vi "PC_Consumer_DMA.vi"() -> ()   [LabVIEW 2019]
uses:
  <vilib>/FPGAPlugInAG/cRIO-9074/niLvFpga_Open_cRIO-9074.vi
  <vilib>/FPGAPlugInAG/cRIO-9074/niLvFpga_Reset_cRIO-9074.vi
  <vilib>/rvi/interface/common/niFpgaWaitOnOcc.vi
  <vilib>/Utility/error.llb/Error Cluster From Error Code.vi
  <vilib>/rvi/errors/niLvFpgaAdjustHostInterfaceError.vi
  <vilib>/FPGAPlugInAG/cRIO-9074/niLvFpga_Run_cRIO-9074.vi
  <vilib>/RVI Host/nirviSupport.llb/nirviErrorClusterFromErrorCode.vi
  FPGA_RW_Vars.vi
  <vilib>/FPGAPlugInAG/cRIO-9074/niLvFpga_Close_cRIO-9074.vi
  <vilib>/rvi/interface/nirviOpenFPGA/nirviOpenFPGA.xnode
  FPGA Bitfiles/bancadaamaciamen_FPGATarget_[FPGA]DeltaSigMa_JyyHRzhCmwA.lvbitx
  FPGA_DAQ_Int.vi
  <vilib>/rvi/interface/nirviMethod/nirviMethod.xnode
  <vilib>/rvi/interface/nirviReadWriteControl/nirviReadWriteControl.xnode
  <vilib>/rvi/interface/nirviCloseFPGA/nirviCloseFPGA.xnode
  <vilib>/rvi/errors/niLvFpgaMergeErrorWithErrorCode.vi
  <vilib>/rvi/interface/nirviMethod/StockFPGA_InlinedMethodWaitForSingleIRQ.vi
  <vilib>/FPGAPlugInAG/cRIO-9074/niLvFpga_WaitOnIrq_cRIO-9074.vi
  <vilib>/FPGAPlugInAG/cRIO-9074/niLvFpga_AcknowledgeIrq_cRIO-9074.vi
  <vilib>/FPGAPlugInAG/cRIO-9074/niLvFpga_ConfigureFifo_cRIO-9074.vi
  <vilib>/FPGAPlugInAG/cRIO-9074/niLvFpga_StartFifo_cRIO-9074.vi
  NiFpgaLv.dll
  <vilib>/FPGAPlugInAG/cRIO-9074/niLvFpga_ReadFifo_cRIO-9074.vi
  <vilib>/FPGAPlugInAG/cRIO-9074/niLvFpga_StopFifo_cRIO-9074.vi
panel:
  out "Vibração + Tensão":waveform(dbl)[](graph)
  in  "Reset Vibracão":bool caption="Reset"
  in  "Reset Tensão":bool caption="Reset"
  out "Gráfico Tensão":waveform(dbl)(graph)
  out "Gráfico Vibração":waveform(dbl)(graph)
  out "Reading?":bool
  out "Calibration Voltage (NI 9225)":cluster{"LSB Weight":dbl, "Offset":dbl}[](array[cluster])
  out "Calibration Vibration (NI 9234)":cluster{"LSB Weight":dbl, "Offset":dbl}[](array[cluster])
  out "Calibration Current (NI 9215)":cluster{"LSB Weight":dbl, "Offset":dbl}[](array[cluster])
  out "Temperature 2 (NI-9219)":T1
  out "Vibration (NI-9234)":cluster{"Vibration (CH1)":waveform(dbl)}
  out "Voltage (NI-9225)":cluster{"Voltage (CH0)":waveform(dbl)}
  out "Voltage (NI-9215)":cluster{"Voltage LEM (CH3)":waveform(dbl)}
  out "Temperature (NI-9219)":T1
  out "Waveform Volt":waveform(dbl)[](graph)
  out "Waveform Cur":waveform(dbl)[](graph)
  in  "ElementsPerCycle":u32=25600
  out "Waveform Vib":waveform(dbl)[](graph)
  out "Configuração realizada":bool
  out "Actual Depth":i32
  out "Requested Depth":i32
  out "Measurements per Cycle":i32
  in  "Stop":bool
  out "Error Out":errorcluster
  # "Configuração"
  # "Leitura"
  # "Sensores de Vibração"
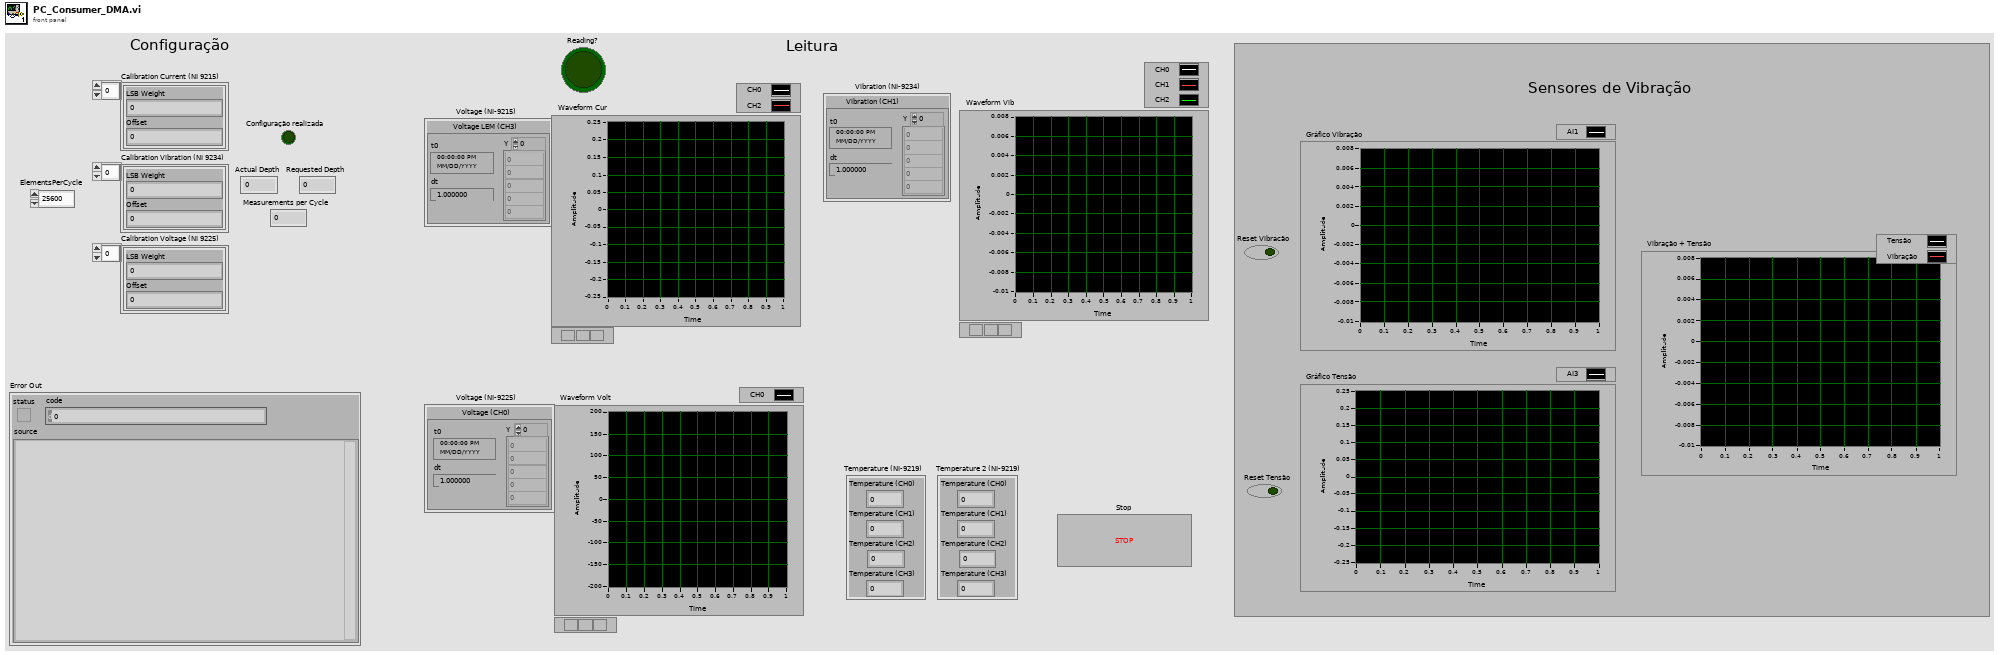
[diagram p1: front panel]
types:
  T1 = cluster{"Temperature (CH0)":dbl, "Temperature (CH1)":dbl, "Temperature (CH2)":dbl, "Temperature (CH3)":dbl}
  T2 = cluster{"Temperature (ºC)":dbl, "Temperature (ºC)":dbl, "Temperature (ºC)":dbl, "Temperature (ºC)":dbl}
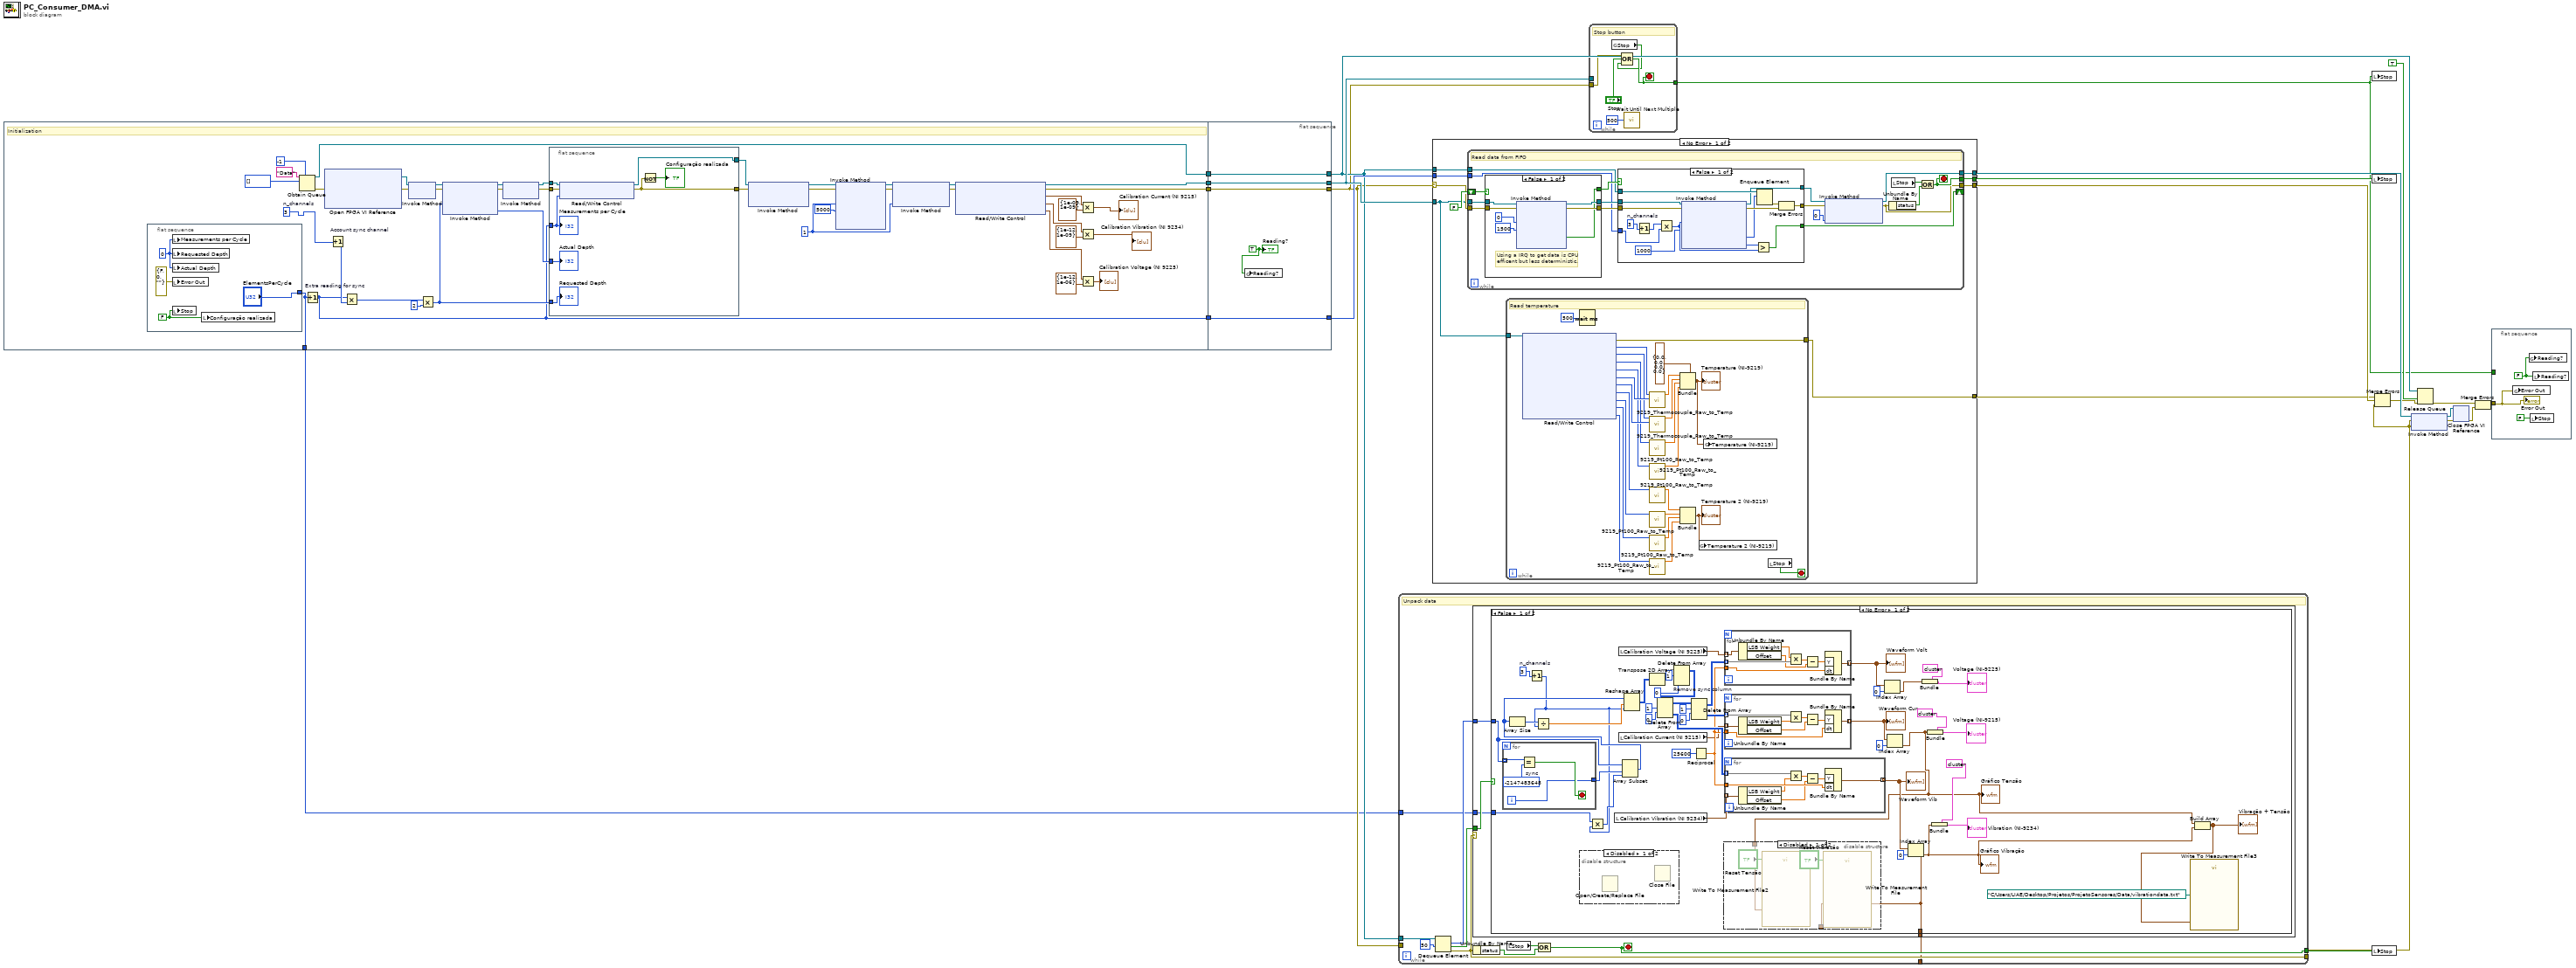
[diagram p0: block diagram]
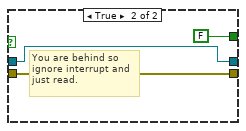
[diagram p6: hidden frame]
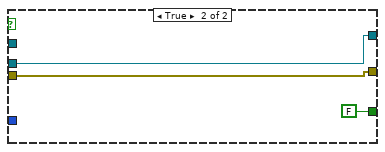
[diagram p7: hidden frame]
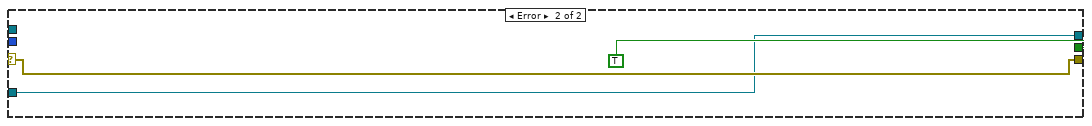
[diagram p8: hidden frame]
diagram:
  n1 = flat-sequence {
    tunnel: [w25] -> w5
    tunnel: [w39] -> w4
    tunnel: [w51] -> w3
    tunnel: [w38] -> w2
    tunnel: [w24] -> w1
    tunnel: [w79] -> w13
    tunnel: [w80] -> w16
    tunnel: [w81] -> w22
    tunnel: [w82] -> w17
    tunnel: w5 -> [w82]
    tunnel: w4 -> [w81]
    tunnel: w3 -> [w80]
    tunnel: w2 -> [w79]
    frame #0 {
      w41 = 1 ("IRQ Number(s)")
      w27 = u32 3  # n_channels
      # "Initialization"
      n2 = flat-sequence {
        tunnel: ["ElementsPerCycle"] -> w24
        frame #0 {
          w75 = 0
          w76 = FALSE ("Stop")
          n3 = local write "Measurements per Cycle"(w75) -> ()
          n4 = local write "Requested Depth"(w75) -> ()
          n5 = local write "Actual Depth"(w75) -> ()
          n6 = local write "Error Out"(errorcluster {"status"=FALSE, "code"=0, "source"=""} ("error constant")) -> ()
          n7 = local write "Stop"(w76) -> ()
          n8 = local write "Configuração realizada"(w76) -> ()
        }
      }
      n9 = Obtain Queue(max queue size (-1, unlimited)=-1, name (unnamed)="Data", element data type=i32[] [] ("Data")) -> (queue out=w51:refnum<queue>, error out=w65:errorcluster)  [unwired: 2 in, 1 out]
      n10 = Increment "Extra reading for sync"(x=w24) -> (x+1=w25:u32)
      n11 = xnode "Open FPGA VI Reference"("error in"=w65) -> ("FPGA VI Reference Out"=w63:refnum<k20>, "error out"=w62:errorcluster)  [unwired: 1 in]
      n12 = Increment "Account sync channel"(x=w27) -> (x+1=w26:u32)
      n13 = Multiply(x=w25, y=w26) -> (x*y=w52:u32)
      n14 = xnode "Invoke Method"("FPGA VI Reference In"=w63, "error in"=w62) -> ("FPGA VI Reference Out"=w49:refnum<k20>, "error out"=w48:errorcluster)
      n15 = Multiply(x=w52, y=u32 2) -> (x*y=w54:u32)
      n16 = xnode "Invoke Method"("FPGA VI Reference In"=w49, "error in"=w48, "Requested Depth"=w54) -> ("FPGA VI Reference Out"=w61:refnum<k20>, "error out"=w60:errorcluster, "Actual Depth"=w53:u32)
      n17 = xnode "Invoke Method"("FPGA VI Reference In"=w61, "error in"=w60) -> ("FPGA VI Reference Out"=w59:refnum<k20>, "error out"=w57:errorcluster)
      n18 = flat-sequence {
        tunnel: w59 -> [w73]
        tunnel: [w72] -> w58
        tunnel: w57 -> [w71]
        tunnel: [w67] -> w56
        tunnel: w25 -> [w70]
        tunnel: w54 -> [w69]
        tunnel: w53 -> [w68]
        frame #0 {
          n19 = xnode "Read/Write Control"("FPGA VI Reference In"=w73, "error in"=w71, "Measurements per cycle"=w70) -> ("FPGA VI Reference Out"=w72:refnum<k20>, "error out"=w67:errorcluster)
          n20 = Not(x=w67) -> (.not. x?=→"Configuração realizada":bool)
          "Measurements per Cycle" <- w70
          "Requested Depth" <- w69
          "Actual Depth" <- w68
        }
      }
      n21 = xnode "Invoke Method"("FPGA VI Reference In"=w58, "error in"=w56) -> ("FPGA VI Reference Out"=w46:refnum<k20>, "error out"=w44:errorcluster)  [unwired: 1 in]
      n22 = xnode "Invoke Method"("FPGA VI Reference In"=w46, "error in"=w44, "IRQ Number(s)"=w41, "Timeout (ms)"=5000) -> ("FPGA VI Reference Out"=w43:refnum<k20>, "error out"=w42:errorcluster)  [unwired: 2 out]
      n23 = xnode "Invoke Method"("FPGA VI Reference In"=w43, "error in"=w42, "IRQ Number(s)"=w41) -> ("FPGA VI Reference Out"=w40:refnum<k20>, "error out"=w37:errorcluster)
      n24 = xnode "Read/Write Control"("FPGA VI Reference In"=w40, "error in"=w37) -> ("FPGA VI Reference Out"=w39:refnum<k20>, "error out"=w38:errorcluster, "Calibration Current (NI 9215)"=w36:cluster{"LSB Weight":u32, "Offset":i32}[], "Calibration Vibration (NI 9234)"=w35:cluster{"LSB Weight":u32, "Offset":i32}[], "Calibration Voltage (NI 9225)"=w34:cluster{"LSB Weight":u32, "Offset":i32}[])
      n25 = Multiply(x=w36, y=cluster{"LSB Weight":dbl, "Offset":dbl} {"LSB Weight"=1e-09, "Offset"=1e-09} ("x*y")) -> (x*y=→"Calibration Current (NI 9215)":cluster{"LSB Weight":dbl, "Offset":dbl}[])
      n26 = Multiply(x=w35, y=cluster{"LSB Weight":dbl, "Offset":dbl} {"LSB Weight"=1e-12, "Offset"=1e-09} ("x*y")) -> (x*y=→"Calibration Vibration (NI 9234)":cluster{"LSB Weight":dbl, "Offset":dbl}[])
      n27 = Multiply(x=w34, y=cluster{"LSB Weight":dbl, "Offset":dbl} {"LSB Weight"=1e-12, "Offset"=1e-06} ("x*y")) -> (x*y=→"Calibration Voltage (NI 9225)":cluster{"LSB Weight":dbl, "Offset":dbl}[])
    }
    frame #1 {
      w78 = TRUE ("Reading?")
      n28 = global write "FPGA_RW_Vars.vi" "Reading?"(w78) -> ()
      "Reading?" <- w78
    }
  }
  n29 = while {
    tunnel: w13 -> [_]
    tunnel: [w85] -> w8
    tunnel: w16 -> [w91]
    tunnel: [w89] -> w14
    tunnel: w1 -> [w84]
    tunnel: [w83] -> _
    stop <- w89 stop-if-true
    # "Unpack data"
    n30 = Dequeue Element(queue=w91, timeout in ms (-1)=50) -> (element=w86:i32[], timed out?=w87:bool, error out=w85:errorcluster)  [unwired: 1 in, 1 out]
    n31 = case shown="No Error" w85 {
      tunnel: w86 -> [w96 _]
      tunnel: w87 -> [w95 _]
      tunnel: w84 -> [w94 _]
      tunnel: [w93 _] -> w83
      frame No Error {
        n32 = case shown="False" w95 {
          tunnel: w96 -> [w115 _]
          tunnel: w94 -> [w106 _]
          tunnel: [w98 _] -> w93
          frame False {
            w108 = u32 3  # n_channels
            n33 = for {
              tunnel: w115 -> [w148] mode=indexing
              tunnel: [w145] -> w110
              i -> [w145]
              stop <- w146 stop-if-true
              w147 = -2147483648  # sync
              n34 = Equal?(x=w148, y=w147) -> (x = y?=w146:bool)
            }
            n35 = Increment(x=w108) -> (x+1=w105:u32)
            n36 = disable-structure shown="Disabled" {
              frame Disabled {
                n37 = Open/Create/Replace File() -> ()  [unwired: 6 in, 3 out]
                n38 = Close File() -> ()  [unwired: 2 in, 2 out]
              }
              frame Enabled {
              }
            }
            n39 = Multiply(x=w106, y=w105) -> (x*y=w107:u32)
            n40 = local read "Calibration Vibration (NI 9234)"() -> (w117:cluster{"LSB Weight":dbl, "Offset":dbl}[])
            n41 = local read "Calibration Voltage (NI 9225)"() -> (w119:cluster{"LSB Weight":dbl, "Offset":dbl}[])
            n42 = local read "Calibration Current (NI 9215)"() -> (w118:cluster{"LSB Weight":dbl, "Offset":dbl}[])
            n43 = Array Subset(array=w115, index=w110, length=w107) -> (w109:i32[])
            n44 = Array Size(array=w109) -> (size(s)=w139:i32)
            n45 = Divide(x=w139, y=w105) -> (x/y=w128:dbl)
            n46 = Reshape Array(w109, w128, w105) -> (w129:i32[][])
            n47 = Transpose 2D Array(2D array=w129) -> (transposed array=w114:i32[][])
            n48 = Delete From Array "Remove sync column"(array=w114, length=1, index (row)=0) -> (array with subset deleted=w111:i32[][])  [unwired: 1 in, 1 out]
            n49 = Delete From Array(array=w111, length=1, index (row)=0) -> (deleted portion=w133:i32[][], array with subset deleted=w136:i32[][])  [unwired: 1 in]
            n50 = Delete From Array(array=w136, length=1, index (row)=0) -> (deleted portion=w132:i32[][], array with subset deleted=w131:i32[][])  [unwired: 1 in]
            n51 = Reciprocal(x=25600) -> (1/x=w130:dbl)
            n52 = for {
              tunnel: w131 -> [w153] mode=indexing
              tunnel: [w156] -> w126 mode=indexing
              tunnel: w130 -> [w155]
              tunnel: w119 -> [w149] mode=indexing
              n53 = Unbundle By Name(w149) -> ("LSB Weight"=w152:dbl, "Offset"=w151:dbl)
              n54 = Multiply(x=w152, y=w153) -> (x*y=w154:dbl[])
              n55 = Subtract(x=w154, y=w151) -> (x-y=w150:dbl[])
              n56 = Bundle By Name("Y"=w150, "dt"=w155) -> (w156:waveform(dbl))  [unwired: 1 in]
            }
            "Waveform Volt" <- w126
            n57 = for {
              tunnel: w132 -> [w162] mode=indexing
              tunnel: [w164] -> w122 mode=indexing
              tunnel: w130 -> [w163]
              tunnel: w118 -> [w159] mode=indexing
              n58 = Unbundle By Name(w159) -> ("LSB Weight"=w158:dbl, "Offset"=w157:dbl)
              n59 = Multiply(x=w162, y=w158) -> (x*y=w161:dbl[])
              n60 = Subtract(x=w161, y=w157) -> (x-y=w160:dbl[])
              n61 = Bundle By Name("Y"=w160, "dt"=w163) -> (w164:waveform(dbl))  [unwired: 1 in]
            }
            "Waveform Cur" <- w122
            n62 = for {
              tunnel: w133 -> [w171] mode=indexing
              tunnel: [w168] -> w120 mode=indexing
              tunnel: w130 -> [w172]
              tunnel: w117 -> [w165] mode=indexing
              n63 = Unbundle By Name(w165) -> ("LSB Weight"=w167:dbl, "Offset"=w166:dbl)
              n64 = Multiply(x=w171, y=w167) -> (x*y=w170:dbl[])
              n65 = Subtract(x=w170, y=w166) -> (x-y=w169:dbl[])
              n66 = Bundle By Name("Y"=w169, "dt"=w172) -> (w168:waveform(dbl))  [unwired: 1 in]
            }
            "Waveform Vib" <- w120
            n67 = Index Array(array=w126, index=0) -> (element=w124:waveform(dbl))
            n68 = Index Array(array=w122, index=0) -> (element=w100:waveform(dbl))
            "Gráfico Tensão" <- w100
            n69 = Index Array(array=w120, index=0) -> (element=w98:waveform(dbl))
            "Gráfico Vibração" <- w98
            n70 = disable-structure shown="Disabled" {
              disable-tunnel: w100 -> [w142 _]
              disable-tunnel: w98 -> [w141 _]
              frame Disabled {
                n71 = call "Write To Measurement File2"("Signals"=w142, "Reset"="Reset Tensão") -> ()  [unwired: 15 in, 3 out]
                n72 = call "Write To Measurement File"("Signals"=w141, "Reset"="Reset Vibracão") -> ()  [unwired: 15 in, 3 out]
              }
              frame Enabled {
              }
            }
            n73 = Bundle(cluster=cluster{"Voltage (CH0)":waveform(dbl)} {"Voltage (CH0)"={"t0"=timestamp(0 s since 1904-01-01), "dt"=1.0, "Y"=[]}} ("Voltage (NI-9225)"), "Voltage (CH0)"=w124) -> (→"Voltage (NI-9225)":cluster{"Voltage (CH0)":waveform(dbl)})
            n74 = Bundle(cluster=cluster{"Voltage LEM (CH3)":waveform(dbl)} {"Voltage LEM (CH3)"={"t0"=timestamp(0 s since 1904-01-01), "dt"=3.90625e-05, "Y"=array[25600 elements]}} ("Voltage (NI-9215)"), "Voltage LEM (CH3)"=w100) -> (→"Voltage (NI-9215)":cluster{"Voltage LEM (CH3)":waveform(dbl)})
            n75 = Bundle(cluster=cluster{"Vibration (CH1)":waveform(dbl)} {"Vibration (CH1)"={"t0"=timestamp(0 s since 1904-01-01), "dt"=3.90625e-05, "Y"=array[25600 elements]}} ("Vibration (NI-9234)"), "Vibration (CH1)"=w98) -> (→"Vibration (NI-9234)":cluster{"Vibration (CH1)":waveform(dbl)})
            n76 = Build Array(w100, w98) -> (w99:waveform(dbl)[])
            "Vibração + Tensão" <- w99
            n77 = call "Write To Measurement File3"("Signals"=w99, "Filename"=path "C:/Users/LIAE/Desktop/Projetos/ProjetoSensores/Data/vibrationdata.txt") -> ()  [unwired: 15 in, 3 out]
          }
          frame True {
          }
        }
      }
      frame Error {
      }
    }
    n78 = Unbundle By Name(w85) -> ("status"=w92:bool)
    n79 = local read "Stop"() -> (w88:bool)
    n80 = Compound Arithmetic op=OR(w88, w92) -> (w89:bool)
  }
  n81 = case shown="No Error" w13 {
    selector: w13 -> [w178 w254]
    tunnel: [w181 w254] -> w7
    tunnel: w22 -> [w174 w252]
    tunnel: [w180 TRUE] -> w15
    tunnel: w17 -> [w177 _]
    tunnel: w16 -> [w176 _]
    tunnel: [w175 w252] -> w19
    tunnel: [w173 _] -> w6
    frame No Error {
      n82 = while {
        tunnel: w178 -> [w213]
        tunnel: [w216] -> w181
        tunnel: w174 -> [w223]
        tunnel: [w210] -> w175
        shift-right: [w220] -> _
        shift-left: FALSE -> [w219]
        tunnel: [w217] -> w180
        tunnel: w177 -> [w212]
        tunnel: w176 -> [w211]
        stop <- w217 stop-if-true
        # "Read data from FIFO"
        n83 = case shown="False" w219 {
          tunnel: w223 -> [w230 w233]
          tunnel: w213 -> [w229 w232]
          tunnel: [w226 w233] -> w222
          tunnel: [w225 w232] -> w221
          tunnel: [w224 FALSE ("Timed Out")] -> w214
          frame False {
            # "Using a IRQ to get data is CPU\nefficent but less deterministic."
            n84 = xnode "Invoke Method"("FPGA VI Reference In"=w230, "error in"=w229, "IRQ Number(s)"=0, "Timeout (ms)"=1500) -> ("FPGA VI Reference Out"=w226:refnum<k20>, "error out"=w225:errorcluster, "Timed Out"=w224:bool)  [unwired: 1 out]
          }
          frame True {
            # "You are behind so\nignore interrupt and\njust read."
          }
        }
        n85 = case shown="False" w214 {
          tunnel: w222 -> [w248 w251]
          tunnel: w221 -> [w247 w249]
          tunnel: [w238 w251] -> w207
          tunnel: [w239 FALSE] -> w220
          tunnel: w212 -> [w237 _]
          tunnel: w211 -> [w246 _]
          tunnel: [w244 w249] -> w208
          frame False {
            w235 = u32 3  # n_channels
            n86 = Increment(x=w235) -> (x+1=w236:u32)
            n87 = Multiply(x=w236, y=w237) -> (x*y=w242:u32)
            n88 = xnode "Invoke Method"("FPGA VI Reference In"=w248, "error in"=w247, "Number of Elements"=w242, "Timeout (ms)"=1000) -> ("FPGA VI Reference Out"=w238:refnum<k20>, "error out"=w245:errorcluster, "Data"=w241:i32[], "Elements Remaining"=w243:u32)
            n89 = Greater? ("Make sure you aren't behind")(x=w243, y=w242) -> (0:w239:bool)
            n90 = Enqueue Element(queue=w246, element=w241) -> (error out=w240:errorcluster)  [unwired: 2 in, 2 out]
            n91 = Merge Errors(w240, w245) -> (w244:errorcluster)
          }
          frame True {
          }
        }
        n92 = xnode "Invoke Method"("FPGA VI Reference In"=w207, "error in"=w208, "IRQ Number(s)"=0) -> ("FPGA VI Reference Out"=w210:refnum<k20>, "error out"=w216:errorcluster)
        n93 = Unbundle By Name(w216) -> ("status"=w218:bool)
        n94 = local read "Stop"() -> (w209:bool)
        n95 = Compound Arithmetic op=OR(w209, w218) -> (w217:bool)
      }
      n96 = while {
        tunnel: w174 -> [w205]
        tunnel: [w201] -> w173
        stop <- w202 stop-if-true
        # "Read temperature"
        n97 = xnode "Read/Write Control"("FPGA VI Reference In"=w205) -> ("error out"=w201:errorcluster, "Temp0"=w203:i32, "Temp1"=w200:i32, "Temp2"=w198:u32, "Temp3"=w197:u32, "CJC0"=w204:u32, "CJC1"=w199:u32, "Temp0 D2"=w191:u32, "Temp1 D2"=w190:u32, "Temp2 D2"=w189:u32, "Temp3 D2"=w188:u32)  [unwired: 1 in, 1 out]
        n98 = Wait (ms)(milliseconds to wait=u32 500) -> ()  [unwired: 1 out]
        n99 = call "9219_Thermocouple_Raw_to_Temp.vi"("CJC0"=w204, "Temp0"=w203) -> ("T"=w195:dbl)  [unwired: 9 in]
        n100 = call "9219_Thermocouple_Raw_to_Temp.vi"("CJC0"=w199, "Temp0"=w200) -> ("T"=w194:dbl)  [unwired: 9 in]
        n101 = call "9219_Pt100_Raw_to_Temp.vi"("Raw Data"=w198) -> ("Temperature (ºC)"=w193:dbl)  [unwired: 10 in]
        n102 = call "9219_Pt100_Raw_to_Temp.vi"("Raw Data"=w197) -> ("Temperature (ºC)"=w192:dbl)  [unwired: 10 in]
        n103 = call "9219_Pt100_Raw_to_Temp.vi"("Raw Data"=w191) -> ("Temperature (ºC)"=w187:dbl)  [unwired: 10 in]
        n104 = call "9219_Pt100_Raw_to_Temp.vi"("Raw Data"=w190) -> ("Temperature (ºC)"=w186:dbl)  [unwired: 10 in]
        n105 = call "9219_Pt100_Raw_to_Temp.vi"("Raw Data"=w189) -> ("Temperature (ºC)"=w185:dbl)  [unwired: 10 in]
        n106 = call "9219_Pt100_Raw_to_Temp.vi"("Raw Data"=w188) -> ("Temperature (ºC)"=w184:dbl)  [unwired: 10 in]
        n107 = Bundle(cluster=T1 {"Temperature (CH0)"=0.0, "Temperature (CH1)"=0.0, "Temperature (CH2)"=0.0, "Temperature (CH3)"=0.0} ("Temperature (NI-9219) 2"), "Temperature (CH0)"=w195, "Temperature (CH1)"=w194, "Temperature (CH2)"=w193, "Temperature (CH3)"=w192) -> (w183:T1)
        "Temperature (NI-9219)" <- w183
        n108 = Bundle("Temperature (ºC)"=w187, "Temperature (ºC)"=w186, "Temperature (ºC)"=w185, "Temperature (ºC)"=w184) -> (w182:T2)  [unwired: 1 in]
        "Temperature 2 (NI-9219)" <- w182
        n109 = global write "FPGA_RW_Vars.vi" "Temperature 2 (NI-9219)"(w182) -> ()
        n110 = global write "FPGA_RW_Vars.vi" "Temperature (NI-9219)"(w183) -> ()
        n111 = local read "Stop"() -> (w202:bool)
      }
    }
    frame Error {
    }
  }
  n112 = while "Debug Loop" {
    tunnel: w22 -> [_]
    tunnel: [w258] -> w12
    tunnel: w13 -> [w257]
    stop <- w258 stop-if-true
    # "Stop button"
    n113 = global read "FPGA_RW_Vars.vi" "Stop"() -> (w255:bool)
    n114 = Compound Arithmetic op=OR(w257, "Stop", w255) -> (w258:bool)
    n115 = call "Wait Until Next Multiple"("Count(mSec)"=u32 500) -> ()  [unwired: 1 out]
  }
  n116 = local write "Stop"(w12) -> ()
  n117 = local write "Stop"(w15) -> ()
  n118 = local write "Stop"(w14) -> ()
  n119 = Merge Errors(w6, w7, w8) -> (w9:errorcluster)
  n120 = xnode "Invoke Method"("FPGA VI Reference In"=w19, "error in"=w8) -> ("FPGA VI Reference Out"=w11:refnum<k20>, "error out"=w10:errorcluster)
  n121 = Release Queue(queue=w16, force destroy? (F)=TRUE, error in (no error)=w9) -> (error out=w21:errorcluster)  [unwired: 2 out]
  n122 = xnode "Close FPGA VI Reference"("FPGA VI Reference In"=w11, "error in"=w10) -> ("error out"=w18:errorcluster)
  n123 = Merge Errors(w21, w18) -> (w23:errorcluster)
  n124 = flat-sequence {
    tunnel: w23 -> [w260]
    tunnel: w12 -> [_]
    frame #0 {
      w261 = FALSE ("Reading?")
      n125 = global write "FPGA_RW_Vars.vi" "Error Out"(w260) -> ()
      n126 = global write "FPGA_RW_Vars.vi" "Reading?"(w261) -> ()
      n127 = local write "Stop"(FALSE ("Stop")) -> ()
      n128 = local write "Reading?"(w261) -> ()
      "Error Out" <- w260
    }
  }
